vi "AuMT8852B EDR Differential Phase Encoding Extended Results LEG.vi"(5 "Stage":T1(ring), 8 "error in (no error)":errorcluster, 11 "VISA session":refnum<visa-resource-name>) -> (0 "error out":errorcluster, 2 "error code":i32, 3 "VISA session out":refnum<visa-resource-name>, 4 "Results":T2)   [LabVIEW 2017]
doc: "Anritsu MT8852B Bluetooth Tester\n\n<B>NOTE:</B> USE THIS VI ONLY FOR MT8852B FIRMWARE VERSIONS UP TO AND INCLUDING 4.08.100\n\nReturns the results of the EDR Differential Phase test.\n\nINPUTS\nStage - results of the individual hopping stages of the test.\n\nOUTPUTS\nResults - measurements made during the test."
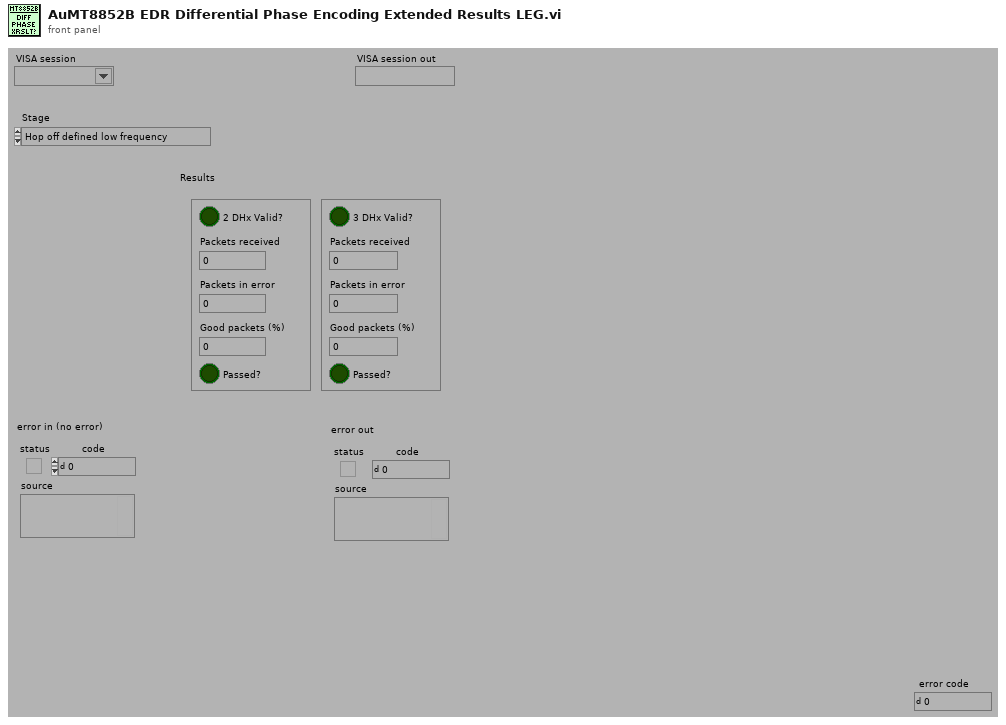
[diagram p1: front panel]
types:
  T1 = enum16{"Hop off defined low frequency", "Hop off defined medium frequency", "Hop off defined high frequency", "Hop on any channels"}
  T2 = cluster{"2 DHx Valid?":bool, "Packets received":u32, "Packets in error":u32, "Passed?":bool, "Good packets (%)":u32, "3 DHx Valid?":bool, "Packets received":u32, "Packets in error":u32, "Passed?":bool, "Good packets (%)":u32}
  T3 = enum16{"Simulate", "Range check", "Cache", "Query instrument status"}
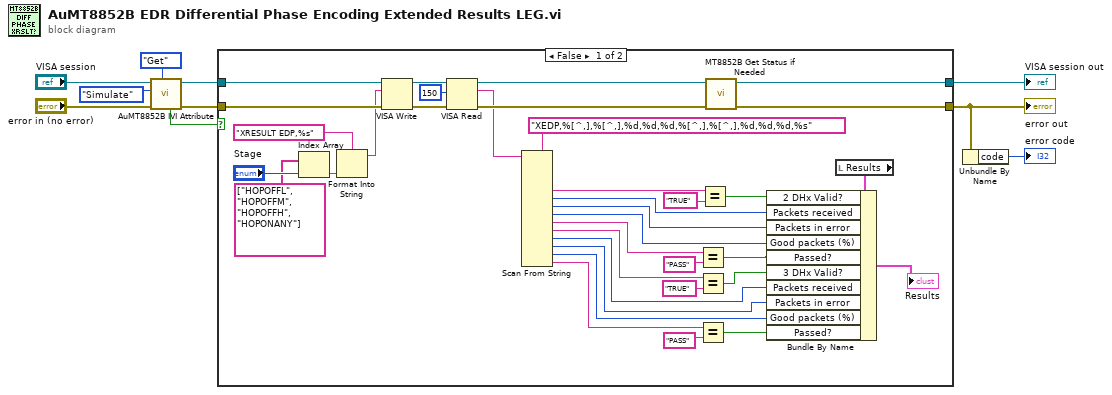
[diagram p0: block diagram]
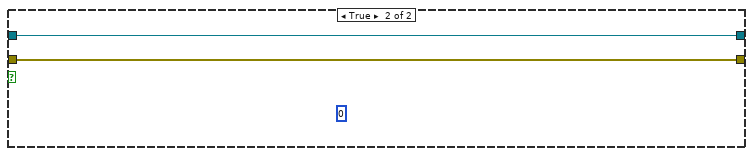
[diagram p2: hidden frame]
diagram:
  n1 = call <instrlib>:"AuMT8852B IVI Attribute.vi"("Set/Get (Set)"=enum16{"Set", "Get"}."Get", "error in (no error)"="error in (no error)", "Flag (Simulate)"=T3."Simulate", "VISA session"="VISA session") -> ("error out"=w7:errorcluster, "VISA session out"=w9:refnum<visa-resource-name>, "Value out"=w3:bool)  [unwired: 5 in]
  n2 = case shown="False" w3 {
    tunnel: [w40 w48] -> w10
    tunnel: [w39 w47] -> w1
    tunnel: w9 -> [w46 w48]
    tunnel: w7 -> [w45 w47]
    frame False {
      n3 = Index Array(array=string[] ["HOPOFFL", "HOPOFFM", "HOPOFFH", "HOPONANY"], index="Stage") -> (element=w26:string)
      n4 = Format Into String(format string="XRESULT EDP,%s" ("write buffer (\"\")"), w26) -> (resulting string=w23:string)  [unwired: 2 in, 1 out]
      n5 = VISA Write(VISA resource name=w46, write buffer=w23, error in (no error)=w45) -> (VISA resource name out=w44:refnum<visa-resource-name>, error out=w43:errorcluster)  [unwired: 1 out]
      n6 = VISA Read(VISA resource name=w44, byte count=u32 150 ("byte count (0)"), error in (no error)=w43) -> (VISA resource name out=w38:refnum<visa-resource-name>, read buffer=w21:string, error out=w37:errorcluster)  [unwired: 1 out]
      n7 = Scan From String(format string="XEDP,%[^,],%[^,],%d,%d,%d,%[^,],%[^,],%d,%d,%d,%s" ("Format String"), input string=w21) -> (output 2=w20:string, output 3=w19:i32, output 4=w18:i32, output 5=w17:i32, output 6=w15:string, output 7=w16:string, output 8=w14:i32, output 9=w13:i32, output 10=w12:i32, output 11=w11:string)  [unwired: 14 in, 3 out]
      n8 = Equal?(x=w15, y="PASS") -> (x = y?=w31:bool)
      n9 = Equal?(x=w16, y="TRUE") -> (x = y?=w30:bool)
      n10 = Equal?(x=w11, y="PASS") -> (x = y?=w29:bool)
      n11 = Equal?(x=w20, y="TRUE") -> (x = y?=w34:bool)
      n12 = call <instrlib>:"MT8852B Get Status if Needed.vi"("error in (no error)"=w37, "VISA session"=w38) -> ("error out"=w39:errorcluster, "VISA session out"=w40:refnum<visa-resource-name>)  [unwired: 8 in]
      n13 = local read "Results"() -> (w35:T2)
      n14 = Bundle By Name(cluster=w35, "2 DHx Valid?"=w34, "Packets received"=w19, "Packets in error"=w18, "Good packets (%)"=w17, "Passed?"=w31, "3 DHx Valid?"=w30, "Packets received"=w14, "Packets in error"=w13, "Good packets (%)"=w12, "Passed?"=w29) -> (→"Results":T2)
    }
    frame True {
      (unwired) u8 0
    }
  }
  "error out" <- w1
  "VISA session out" <- w10
  n15 = Unbundle By Name(w1) -> ("code"=→"error code":i32)
